vi "Third stepf heating with process.vi"(0 "Arduino Resource In":T1={"VISA resource"="", "Board Type"=enum."Uno", "Connection Type"=enum."USB / Serial", "Bytes Per Packet (15)"=15}, 1 "Shift left":i32, 7 "Boolean from second step":bool, 11 "Error In":errorcluster, 12 "Температура после shift register":dbl[](array[numeric])) -> (3 "Shift right":i32, 4 "Arduino Resource Out":T1={"VISA resource"="", "Board Type"=enum."Uno", "Connection Type"=enum."USB / Serial", "Bytes Per Packet (15)"=15}, 14 "Текущая температура":dbl[](array[numeric]), 15 "Error Out":errorcluster)   [LabVIEW 2016]
uses:
  <vilib>/LabVIEW Interface for Arduino/Type Defs/Arduino Resource.ctl
  <vilib>/LabVIEW Interface for Arduino/Type Defs/Board Type.ctl
  <vilib>/LabVIEW Interface for Arduino/LabVIEW Interface for Arduino.lvlib
panel:
  in  "Кол-во погружений в каждый стакан":i32[](array[numeric])=[1, 1, 1, 1]
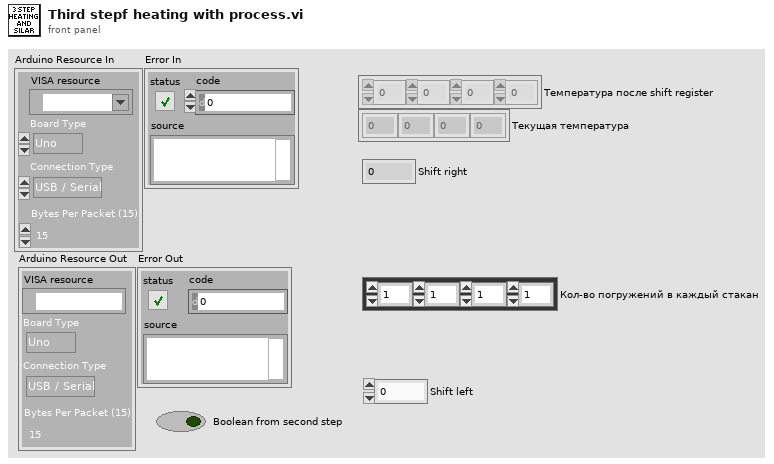
[diagram p1: front panel]
types:
  T1 = typedef "LabVIEW Interface for Arduino.lvlib/Arduino Resource.ctl" = cluster{"VISA resource":refnum<visa-resource-name>, "Board Type":T2, "Connection Type":enum8{"USB / Serial"}, "Bytes Per Packet (15)":u8}
  T2 = typedef "LabVIEW Interface for Arduino.lvlib/Board Type.ctl" = enum16{"Uno", "Dimuelanove w/Atmega 328", "Mega 2560"}
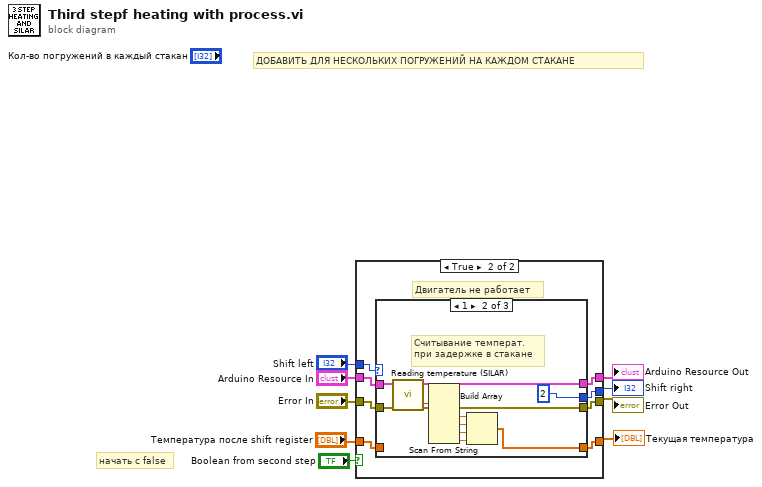
[diagram p0: block diagram]
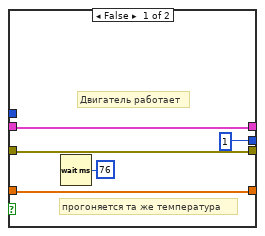
[diagram p2: hidden frame]
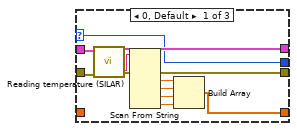
[diagram p3: hidden frame]
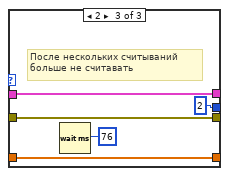
[diagram p4: hidden frame]
diagram:
  # "начать с false"
  # "ДОБАВИТЬ ДЛЯ НЕСКОЛЬКИХ ПОГРУЖЕНИЙ НА КАЖДОМ СТАКАНЕ"
  n1 = case shown="True" "Boolean from second step" {
    tunnel: [w10 w15] -> w9
    tunnel: [w12 w17] -> w8
    tunnel: "Arduino Resource In" -> [w10 w21]
    tunnel: "Error In" -> [w12 w20]
    tunnel: "Shift left" -> [_ w22]
    tunnel: [1 w16] -> w4
    tunnel: [w13 w18] -> w1
    tunnel: "Температура после shift register" -> [w13 w19]
    frame False {
      # "прогоняется та же температура"
      # "Двигатель работает"
      n2 = Wait (ms)(milliseconds to wait=u32 76) -> ()  [unwired: 1 out]
    }
    frame True {
      # "Двигатель не работает"
      n3 = case shown="1" w22 {
        selector: w22 -> [w28 _ _]
        tunnel: [w33 w41 w48] -> w15
        tunnel: [w31 w40 w47] -> w17
        tunnel: w21 -> [w30 w43 w48]
        tunnel: w20 -> [w29 w42 w47]
        tunnel: [w28 2 2] -> w16
        tunnel: [w23 w39 w45] -> w18
        tunnel: w19 -> [_ _ w45]
        frame 0, Default {
          n4 = call "Reading temperature (SILAR).vi"("error in"=w29, "Arduino Resource in"=w30) -> ("error out"=w31:errorcluster, "Arduino Resource"=w33:T1, "read buffer"=w32:string)  [unwired: 7 in]
          n5 = Scan From String(input string=w32, error in=w31) -> (output 1=w27:dbl, output 2=w26:dbl, output 3=w25:dbl, output 4=w24:dbl)  [unwired: 6 in, 3 out]
          n6 = Build Array(w27, w26, w25, w24) -> (w23:dbl[])
        }
        frame 1 {
          # "Считывание температ.\nпри задержке в стакане"
          n7 = call "Reading temperature (SILAR).vi"("error in"=w42, "Arduino Resource in"=w43) -> ("error out"=w40:errorcluster, "Arduino Resource"=w41:T1, "read buffer"=w44:string)  [unwired: 7 in]
          n8 = Scan From String(input string=w44, error in=w40) -> (output 1=w38:dbl, output 2=w37:dbl, output 3=w36:dbl, output 4=w35:dbl)  [unwired: 6 in, 3 out]
          n9 = Build Array(w38, w37, w36, w35) -> (w39:dbl[])
        }
        frame 2 {
          # "После нескольких считываний\nбольше не считавать"
          n10 = Wait (ms)(milliseconds to wait=u32 76) -> ()  [unwired: 1 out]
        }
      }
    }
  }
  "Arduino Resource Out" <- w9
  "Error Out" <- w8
  "Shift right" <- w4
  "Текущая температура" <- w1
